vi "Correct IMU Bearing.vi"(1 "Read Bearing":dbl, 2 "Bearing modification":dbl[](graph)) -> (0 "Actual Bearing":dbl)   [LabVIEW 2011]
uses:
  <vilib>/Analysis/coordinate.llb/Angle Units.ctl
  <vilib>/Analysis/coordinate.llb/Angle Range (Degree).ctl
  <vilib>/Analysis/coordinate.llb/Wrap Angle (scalar).vi
  <vilib>/Analysis/NI_AAL_Angle.lvlib
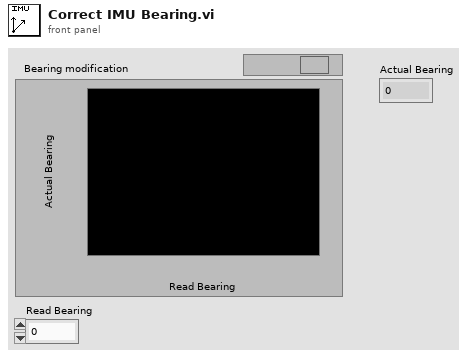
[diagram p1: front panel]
types:
  T1 = typedef "NI_AAL_Angle.lvlib/Angle Range (Degree).ctl" = u16
  T2 = typedef "NI_AAL_Angle.lvlib/Angle Units.ctl" = i32
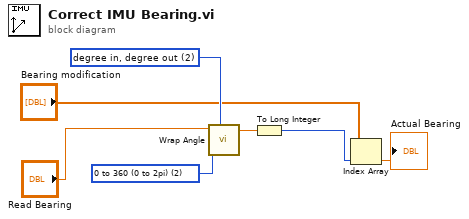
[diagram p0: block diagram]
diagram:
  w6 = T1 2 items=["none", "-180 to 180 (-pi to pi)", "0 to 360 (0 to 2pi)"] ("angle range")
  w7 = T2 2 items=["radian in, radian out", "radian in, degree out", "degree in, degree out", "degree in, radian out"] ("angle units")
  n1 = call-poly <vilib>:"Wrap Angle.vi"("angle units"=w7, "angle range"=w6, "angle in"="Read Bearing") -> ("angle out"=w4:dbl)  [unwired: 7 in, 1 out]
  n2 = To Long Integer(number=w4) -> (32bit integer=w3:i32)
  n3 = Index Array(array="Bearing modification", index=w3) -> (element=→"Actual Bearing":dbl)
